vi "GenerateBurst.vi"(8 "error in (no error)":errorcluster, 9 "Burst mode":T1, 11 "reference in":refnum<class "niMmWave_Transceiver.lvclass">) -> (0 "error out":errorcluster, 3 "reference out":refnum<class "niMmWave_Transceiver.lvclass">)   [LabVIEW 2019, in "niMmWave_Transceiver.lvclass"]
doc: "Generates single burst"
uses:
  niMmWave_Transceiver.lvclass
  C:/Barkhausen mmWave radar/Development/modules/mmw_instrument/src_LabVIEW/Host/SubVIs/mmWave instrument_class/mmWave instrument.lvclass
  mmWave instrument_class/BurstMode.ctl
  mmWave HW Control/HW custom error.ctl
  mmWave instrument_class/Instrument state.ctl
  Low-level/TypeDefs/Direction.ctl
  mmWave HW Control/mmWave HW Control.lvlib
  FPGA sequener API/FPGA sequencer API.lvlib
  mmWave instrument_class/mmWave instrument.lvclass
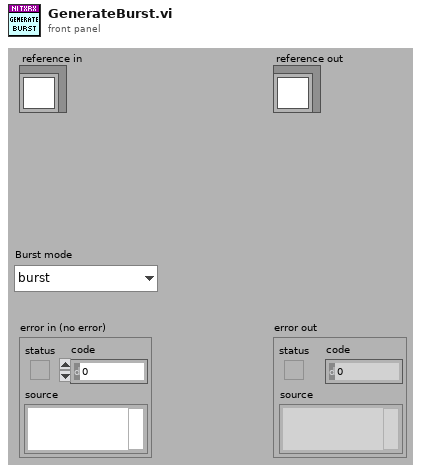
[diagram p1: front panel]
types:
  T1 = typedef "mmWave instrument.lvclass/BurstMode.ctl" = enum16{"burst", "continuous"}
  T2 = typedef "mmWave instrument.lvclass/Instrument state.ctl" = enum16{"Off", "Initialization", "Configuration", "Running", "Calibration"}
  T3 = typedef "Direction.ctl" = enum16{"Transceiver", "Receiver", "Transmitter"}
  T4 = cluster{"start addr":u32, "end addr":u32, "repeat":u64}
  T5 = typedef "mmWave HW Control.lvlib/HW custom error.ctl" = u16
  T6 = typedef "niMmWave_Transceiver.lvclass/ObjectAttributesRef.ctl" = refnum<data-value>
  T7 = typedef "niMmWave_Transceiver.lvclass/ObjectAttributes.ctl" = cluster{"session":T8[], "HW.RX resources":T21, "RF config":T22, "RX trigger options":T23, "TX trigger options":T23, "RX samples":i32, "Downloaded Bursts":map{string, T26}, "TX Fs":dbl, "RX Fs":dbl, "burst sequence":string[]}
  T8 = typedef "Session.ctl" = cluster{"3620 session":refnum<queue>, "tx baseband session":T9, "rx baseband session":T17, "tx gain (dB)":dbl, "rx gain (dB)":dbl, "hardware configuration":T18, "gain ranging":T19[], "pxi trigger bus information":T20}
  T9 = typedef "Tx Baseband Session.ctl" = cluster{"3610 session":T10, "7902 reference":T16}
  T10 = typedef "ni3610_and_ni3630_Driver_Lib.lvlib/Main Settings.ctl" = cluster{"VISA resource name":refnum<visa-resource-name>, "Address Space":T11, "window_offset":u32, "register_addresses":T12, "required_MM_fpga_version":cluster{"signature":u32, "hardware":u32, "current revision":u32, "oldest revision":u32}, "CPLD Oldest Compat Version ":cluster{"hardware":u32, "CPLD firmware":u32}, "MM_FPGA_image_location":string, "is_init":bool, "card_type":T13, "DacLmkConfigFileName":string, "AdcLmkConfigFileName":string, "AdcConfigFileName":string, "DacConfigFileName_RevA":string, "DacConfigFileName_RevB":string, "Mulde hardware revision":u8, "bypass DAC PLL\n":bool, "IQ Card Revision":T14, "board capability":T15}
  T11 = typedef "VISA Register Access Address Space.ctl" = u16
  T12 = typedef "ni3610_and_ni3630_Driver_Lib.lvlib/Register Adresses.ctl" = cluster{"MM based Registers":cluster{"Revision":u32, "OldestCompatRev":u32, "signature":u32, "scratch":u32, "LedControl":u32, "BoardHwRev":u32, "BoardControl":u32, "ThermalStatus":u32, "BasebandStatus":u32, "BasebandControl":u32, "BasebandAuxSetup":u32, "BasebandAuxStatus":u32, "LmkSyncOutSetup":u32, " AdcSyncOutSetup":u32, " InjSyncOutSetup":u32, " PxiTrig0OutSetup":u32, " PxiTrig1OutSetup":u32, " PxiTrig2OutSetup":u32, " PxiTrig3OutSetup":u32, " PxiTrig4OutSetup":u32, " PxiTrig5OutSetup":u32, " PxiTrig6OutSetup":u32, " PxiTrig7OutSetup":u32}, "CPLD based Registers":cluster{"SlaveSignature":u32, "SlaveRevision":u32, "SlaveOldestCompatRev":u32, "SlaveScratch":u32, "SlaveSetup":u32, "SlaveStatus":u32, "IDacReg_offset":u32, "LMKRegGrp0_offset":u32, "QDacReg_offset":u32, "BrdTempSensorVal":u32, "TempSensorPowerDown":u32, "GPIOReg_offset":u32, "IAdcReg_offset":u32, "QAdcReg_offset":u32, "LMKRegGrp1_offset":u32, "QadcTempSensorVal":u32, "IadcTempSensorVal":u32, "RevisionReg":u32, "VcxoReg":u32, "CpldStatusReg":u32, "PowerReg":u32, "VBiasEnReg":u32, "ExtRefOeReg":u32, "QdacCtrlReg":u32, "QdacStatusReg":u32, "IdacCtrlReg":u32, "IdacStatusReg":u32, "QdacJtagIn":u32, "QdacJtagOut":u32, "IdacJtagIn":u32, "IdacJtagOut":u32, "IqDcSetupReg":u32, "QadcStatusReg":u32, "IadcStatusReg":u32, "BrdSetupReg":u32, "IqDcRevisionReg":u32, "PllStatusReg":u32, "EndpointScratchReg":u32, "AdcSyncCfgReg":u32, "IqCardOpampReg":u32}, "CPLD Register Offset":u32, "MM  Register Offset":u32, " PxiTrig0OutSetup":u32}
  T13 = typedef "ni3610_and_ni3630_Driver_Lib.lvlib/Base Card Type.ctl" = enum16{"unspecified", "ADC", "DAC"}
  T14 = typedef "ni3610_and_ni3630_Driver_Lib.lvlib/IQ Card Revision.ctl" = enum16{"RevA", "RevB", "RevC", "RevD"}
  T15 = typedef "ni3610_and_ni3630_Driver_Lib.lvlib/Board Capability.ctl" = cluster{"baseband sync":enum16{"no baseband sync", "baseband sync"}}
  T16 = typedef "Blank FPGA Reference.ctl" = refnum<k20>
  T17 = typedef "Rx Baseband Session.ctl" = cluster{"3630 session":T10, "7902 reference":T16}
  T18 = typedef "Hardware Configuration.ctl" = cluster{"direction":T3, "baseband only":bool}
  T19 = typedef "Gain Ranging.ctl" = cluster{"gain ranging active scope":string, "gain ranging stream session":refnum<k20>}
  T20 = typedef "PXI Trigger Bus Info.ctl" = cluster{"chassis resource name":refnum<visa-resource-name>, "7902R (TX)":i16, "3610 (TX)":i16, "3620 (IF)":i16, "3630 (RX)":i16, "7902R (RX)":i16}
  T21 = typedef "mmWave HW Control.lvlib/HW TXRX resources cluster.ctl" = cluster{"TX_DAC":refnum<visa-resource-name>, "TX_FPGA":tag, "IF":tag, "RX_ADC":refnum<visa-resource-name>, "RX_FPGA":tag}
  T22 = typedef "mmWave HW Control.lvlib/HW TXRX RF config cluster.ctl" = cluster{"TX.Frequency":dbl, "TX.Gain":dbl, "TX.mmWave adapter":string, "RX.Frequency":dbl, "RX.Gain":dbl, "RX.mmWave adapter":string}
  T23 = typedef "TX trigger config.ctl" = cluster{"delay":dbl, "trig source":T24, "PXI src":i32, "export":T25, "PXI dest":i32}
  T24 = typedef "FPGA Utility.lvlib/FPGA driver trigger source.ctl" = enum16{"Use Tclk", "PXI_Trig", "Aurora RX trig"}
  T25 = typedef "FPGA Utility.lvlib/FPGA driver trigger destination.ctl" = enum16{"None", "Source trig", "Synced trig", "Delayed sync"}
  T26 = typedef "niMmWave_Transceiver.lvclass/BurstInfo.ctl" = cluster{"starting addr":u32, "end addr":u32}
  T27 = typedef "FPGA sequencer API.lvlib/FPGA sequencer ref.ctl" = refnum<k20>
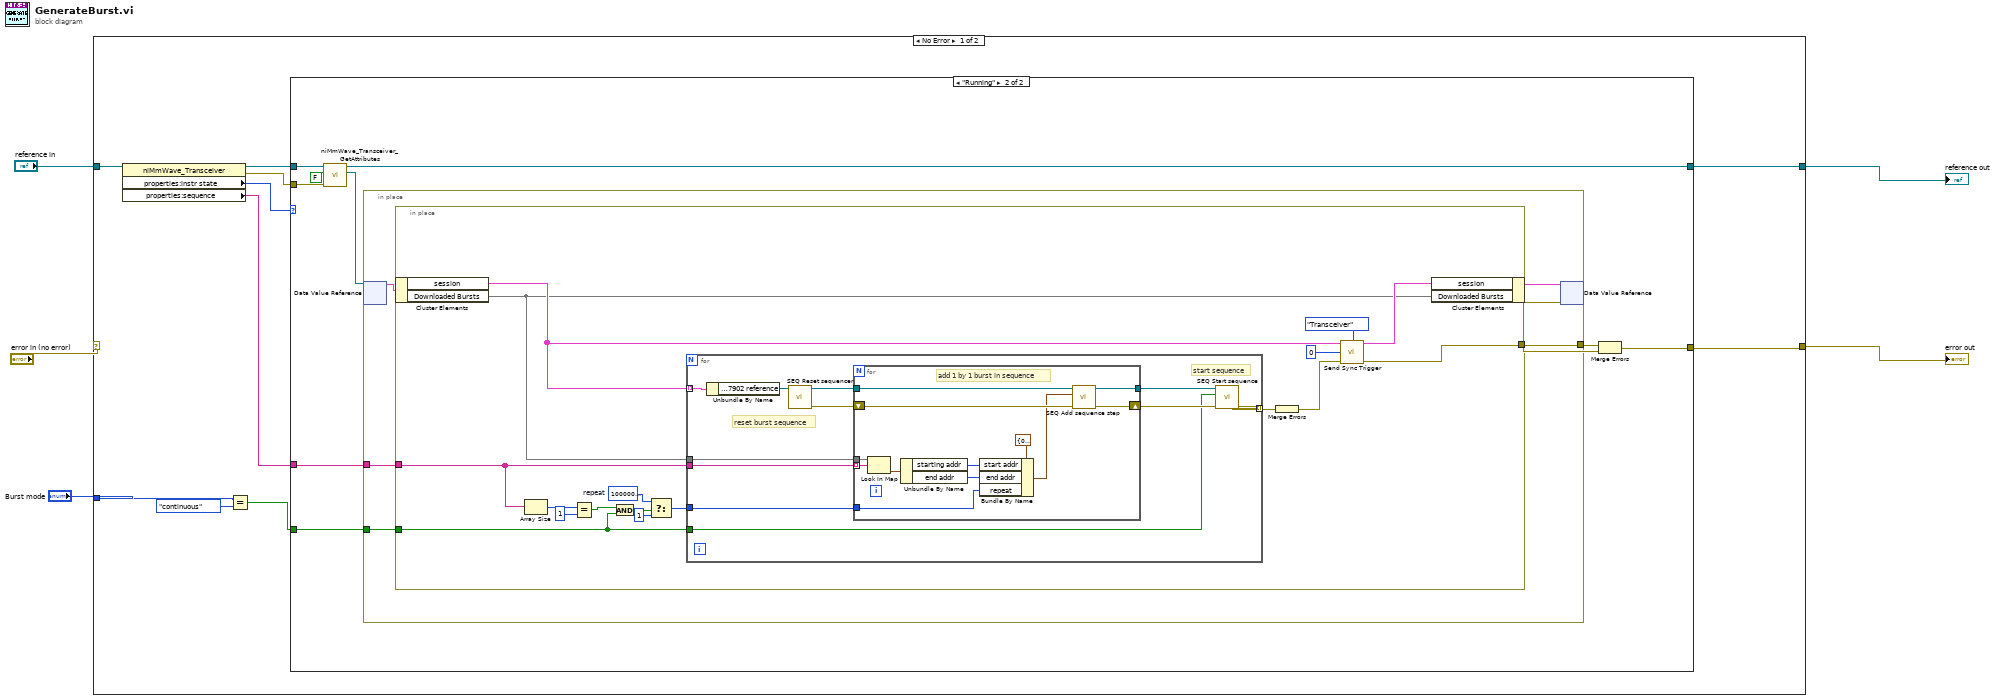
[diagram p0: block diagram]
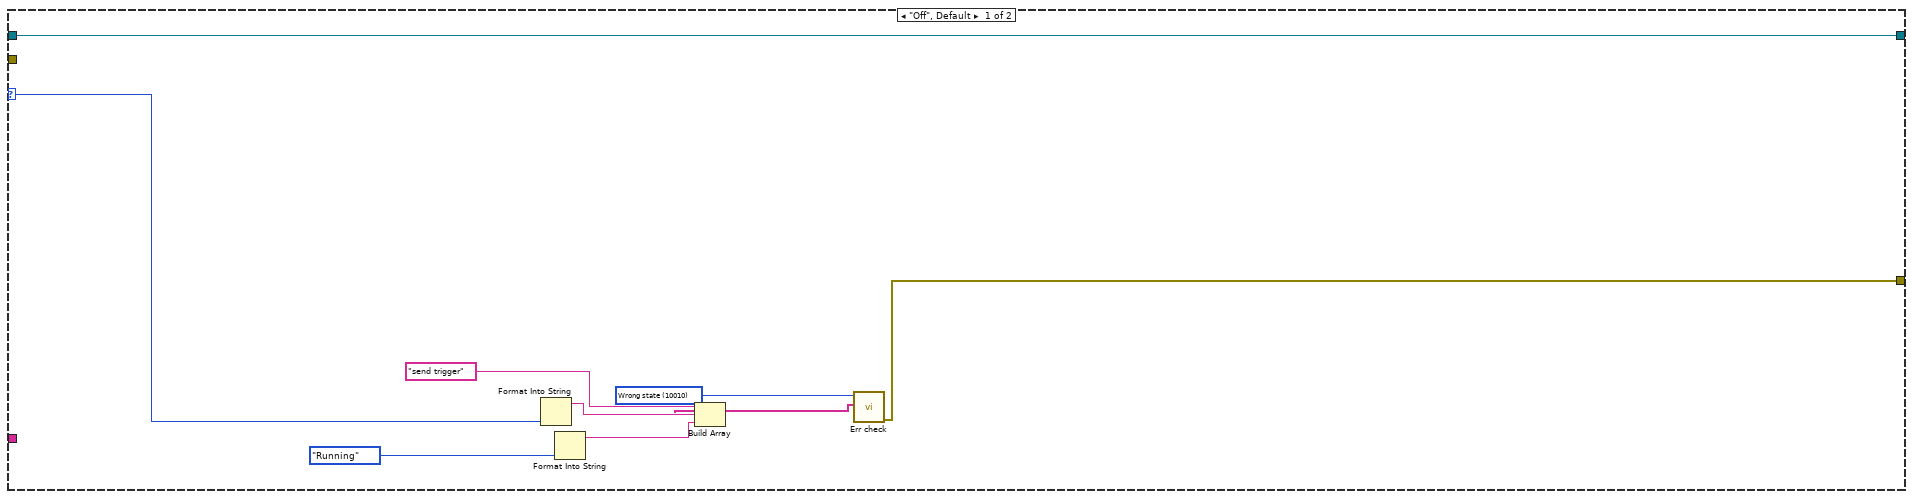
[diagram p2: hidden frame]
diagram:
  n1 = case shown="No Error" "error in (no error)" {
    selector: "error in (no error)" -> [_ w81]
    tunnel: [w10 w81] -> w4
    tunnel: [w14 w80] -> w2
    tunnel: "reference in" -> [w15 w80]
    tunnel: "Burst mode" -> [w9 _]
    frame No Error {
      n2 = property class="niMmWave_Transceiver"(reference=w15) -> (reference out=w13:refnum<class "niMmWave_Transceiver.lvclass">, error out=w12:errorcluster, "properties:instr state"=w11:T2, "properties:sequence"=w6:string[])  [unwired: 1 in]
      n3 = Equal?(x=w9, y=BurstMode."continuous") -> (x = y?=w7:bool)
      n4 = case shown="\"Running\"" w11 {
        selector: w11 -> [w17 _]
        tunnel: [w24 w33] -> w14
        tunnel: w13 -> [w24 w31]
        tunnel: w12 -> [_ w30]
        tunnel: [w16 w27] -> w10
        tunnel: w7 -> [_ w26]
        tunnel: w6 -> [_ w25]
        frame "Off", Default {
          w23 = T5 10010 items=["TX list"=10000, "TX length"=10001, "RX length"=10002, "Fs"=10003, "RF Fc"=10004, "Wrong state"=10010] ("HW custom err")
          n5 = Format Into String(w17) -> (resulting string=w21:string)  [unwired: 3 in, 1 out]
          n6 = Format Into String(Instrument_state."Running" ("properties:instr state")) -> (resulting string=w18:string)  [unwired: 3 in, 1 out]
          n7 = Build Array("send trigger", w21, w18) -> (w20:string[])
          n8 = call "Err check.vi"("Variant Control"=w20, "HW custom err"=w23) -> ("error out"=w16:errorcluster)  [unwired: 9 in]
        }
        frame "Running" {
          n9 = call "niMmWave_Transceiver_GetAttributes.vi"("error in (no error)"=w30, "return data? (T)"=FALSE, "reference in"=w31) -> ("attributes ref"=w32:T6, "reference out"=w33:refnum<class "niMmWave_Transceiver.lvclass">)  [unwired: 5 in, 2 out]
          n10 = in-place {
            in-place-border: [w37] -> w28
            in-place-border: w26 -> [w36]
            in-place-border: w25 -> [w35]
            n11 = in-place-dvr #1(w32) -> (w38:T7)  [unwired: 1 out]
            n12 = in-place {
              in-place-border: [w50] -> w37
              in-place-border: w36 -> [w45]
              in-place-border: w35 -> [w40]
              w43 = u64 1000000000000  # repeat
              n13 = in-place-cluster #2(w38) -> ("session"=w52:T8[], "Downloaded Bursts"=w49:map{string, T26})
              n14 = Array Size(array=w40) -> (size(s)=w48:i32)
              n15 = Equal?(x=w48, y=1) -> (x = y?=w46:bool)
              n16 = And(x=w46, y=w45) -> (x .and. y?=w44:bool)
              n17 = Select(t=w43, s=w44, f=u64 1) -> (s? t:f=w41:u64)
              n18 = for {
                tunnel: w52 -> [w67] mode=indexing
                tunnel: [w65] -> w54 mode=indexing
                tunnel: w45 -> [w60]
                tunnel: w40 -> [w59]
                tunnel: w49 -> [w58]
                tunnel: w41 -> [w57]
                # "start sequence"
                # "reset burst sequence"
                n19 = Unbundle By Name(w67) -> ("tx baseband session.7902 reference"=w66:T16)
                n20 = call "SEQ Reset sequencer.vi"("Refnum in"=w66) -> ("error out"=w63:errorcluster, "Refnum out"=w64:T27)  [unwired: 9 in]
                n21 = for {
                  tunnel: w64 -> [w79]
                  tunnel: [w75] -> w61
                  tunnel: w59 -> [w71] mode=indexing
                  tunnel: w58 -> [w70]
                  shift-right: [w76] -> w62
                  shift-left: w63 -> [w78]
                  tunnel: w57 -> [w68]
                  # "add 1 by 1 burst in sequence"
                  n22 = Look In Map(map=w70, key=w71) -> (value=w69:T26)  [unwired: 1 in, 1 out]
                  n23 = Unbundle By Name(w69) -> ("starting addr"=w73:u32, "end addr"=w72:u32)
                  n24 = Bundle By Name(cluster=T4 {"start addr"=0, "end addr"=299, "repeat"=1} ("seq.new step"), "start addr"=w73, "end addr"=w72, "repeat"=w68) -> (w77:T4)
                  n25 = call "SEQ Add sequence step.vi"("error in (no error)"=w78, "seq.new step"=w77, "Refnum in"=w79) -> ("error out"=w76:errorcluster, "Refnum out"=w75:T27)  [unwired: 7 in]
                }
                n26 = call "SEQ Start sequence.vi"("error in (no error)"=w62, "sequence.cont"=w60, "Refnum in"=w61) -> ("error out"=w65:errorcluster)  [unwired: 7 in, 1 out]
              }
              n27 = Merge Errors(w54) -> (w53:errorcluster)
              n28 = call "Send Sync Trigger.vi"("session in"=w52, "sync select"=Direction."Transceiver", "master device index"=0, "error in"=w53) -> ("session out"=w51:T8[], "error out"=w50:errorcluster)  [unwired: 10 in]
              n29 = in-place-cluster #2("session"=w51, "Downloaded Bursts"=w49) -> (w39:T7)
            }
            n30 = in-place-dvr #1(w39) -> (w29:errorcluster)  [unwired: 1 out]
          }
          n31 = Merge Errors(w28, w29) -> (w27:errorcluster)
        }
      }
    }
    frame Error {
    }
  }
  "error out" <- w4
  "reference out" <- w2
